vi "DAQEG_Get Waveform By Channel.vi"(8 "error in (no error)":errorcluster, 10 "DAQ Channel":string="Dev1/ai0") -> (0 "error out":errorcluster, 2 "waveform":waveform(dbl))   [LabVIEW 2016]
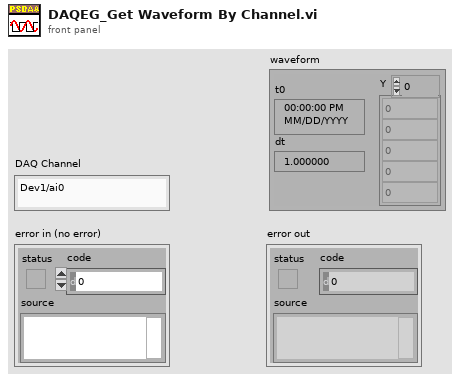
[diagram p1: front panel]
types:
  T1 = cluster{"Queue Name":string, "DAQ Channels":string[], "Queue Type":string}[]
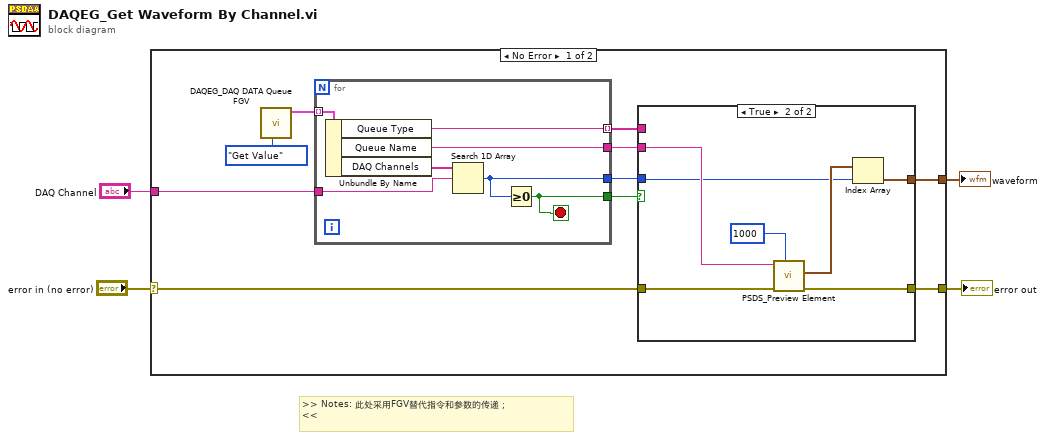
[diagram p0: block diagram]
diagram:
  # ">> Notes: 此处采用FGV替代指令和参数的传递；\n<<"
  n1 = case shown="No Error" "error in (no error)" {
    selector: "error in (no error)" -> [w6 w30]
    tunnel: "DAQ Channel" -> [w14 _]
    tunnel: [w13 w30] -> w3
    tunnel: [w9 _] -> w2
    frame No Error {
      n2 = call "DAQEG_DAQ DATA Queue FGV.vi"("Command"=enum16{"Initialize", "Get Value", "Set Value"}."Get Value") -> ("DAQ DATA Out"=w7:T1)  [unwired: 9 in, 1 out]
      n3 = for {
        tunnel: w7 -> [w29] mode=indexing
        tunnel: w14 -> [w27]
        tunnel: [w26] -> w12
        tunnel: [w25] -> w10
        tunnel: [w24] -> w11
        tunnel: [w23] -> w5 mode=indexing
        stop <- w24 stop-if-true
        n4 = Unbundle By Name(w29) -> ("Queue Type"=w23:string, "Queue Name"=w26:string, "DAQ Channels"=w28:string[])
        n5 = Search 1D Array(1D array=w28, element=w27) -> (index of element=w25:i32)  [unwired: 1 in]
        n6 = Greater Or Equal To 0?(x=w25) -> (x >= 0?=w24:bool)
      }
      n7 = case shown="True" w11 {
        tunnel: w6 -> [w15 w22]
        tunnel: [w15 w21] -> w13
        tunnel: w12 -> [_ w20]
        tunnel: w10 -> [_ w18]
        tunnel: [_ w17] -> w9
        tunnel: w5 -> [_ _]
        frame False {
        }
        frame True {
          n8 = call "PSDS_Preview Element.vi"("Time Out(-1)"=1000, "error in (no error)"=w22, "Object Name"=w20) -> ("error out"=w21:errorcluster, "Wave"=w19:waveform(dbl)[])  [unwired: 6 in, 1 out]
          n9 = Index Array(array=w19, index=w18) -> (element=w17:waveform(dbl))
        }
      }
    }
    frame Error {
    }
  }
  "error out" <- w3
  "waveform" <- w2
